vi "Initialize.vi"(8 "error in":errorcluster, 11 "cCRD Subject in":refnum<class "cCRD Subject.lvclass">) -> (0 "error out":errorcluster, 2 "DVR":refnum<data-value>, 3 "cCRD Subject out":refnum<class "cCRD Subject.lvclass">)   [LabVIEW 2015, in "cCRD Subject.lvclass"]
doc: "This VI must be overridden to provide useful feedback but the parent will provide a reference for a stop occurrence that can be used by the children. Children should provide a reference to the proper data object (loading it into the subject class). The specific data object must be downcasted to the generic data object."
uses:
  cCRD Subject.lvclass
  Reusable/Data/Data.lvclass
  CRDS/Data/cCRDS Data.lvclass
  Reusable/Observer/Data Subject.lvclass/Data Subject.ctl
  Reusable/Observer/Data Subject.lvclass
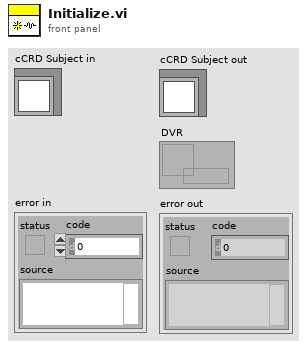
[diagram p1: front panel]
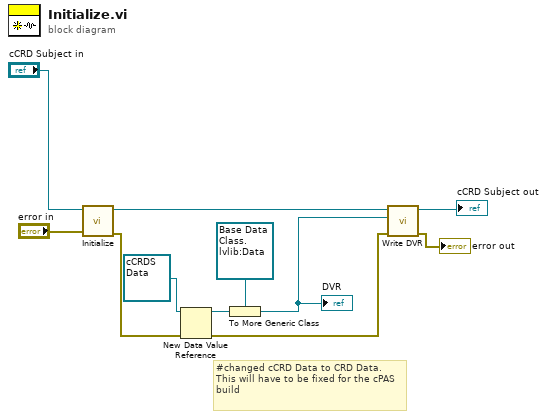
[diagram p0: block diagram]
diagram:
  # "#changed cCRD Data to CRD Data.  This will have to be fixed for the cPAS build"
  n1 = call-parent "Initialize.vi"("error in"="error in", "Data Subject in"="cCRD Subject in") -> ("error out"=w8:errorcluster, "Data Subject out"=w7:refnum<class "cCRD Subject.lvclass">)  [unwired: 7 in, 1 out]
  n2 = New Data Value Reference(data value=refnum<class "cCRDS Data.lvclass"> refnum ("cCRDS Data"), error in=w8) -> (data value reference=w10:refnum<data-value>, error out=w9:errorcluster)
  n3 = To More Generic Class(target class=refnum<data-value> refnum ("data value reference"), reference=w10) -> (generic class reference=w5:refnum<data-value>)
  "DVR" <- w5
  n4 = call "Write DVR.vi"("error in"=w9, "DVR"=w5, "Data Subject in"=w7) -> ("error out"=→"error out":errorcluster, "Data Subject out"=→"cCRD Subject out":refnum<class "cCRD Subject.lvclass">)  [unwired: 7 in]
